vi "Editor Daten auslesen (Sub.vi).vi"(0 "Daten":string, 1 "Formatierung+Namen":string="%d", 2 "Modulname":string, 5 "Zykluslängen Namen":string) -> (6 "Zykluslänge 1":dbl, 7 "Zykluslänge 2":dbl, 8 "1":dbl[][](array[numeric]), 9 "10":dbl[][](array[numeric]), 10 "Z 1":string, 11 "Z 10":string, 12 "2":dbl[][](array[numeric]), 13 "9":dbl[][](array[numeric]), 14 "Z 2":string, 15 "Z 9":string, 16 "3":dbl[][](array[numeric]), 17 "8":dbl[][](array[numeric]), 18 "Z 3":string, 19 "Z 8":string, 20 "4":dbl[][](array[numeric]), 21 "Z 4":string, 22 "5":dbl[][](array[numeric]), 23 "Z5":string, 24 "6":dbl[][](array[numeric]), 25 "Z 6":string, 26 "7":dbl[][](array[numeric]), 27 "Z 7":string)   [LabVIEW 2010]
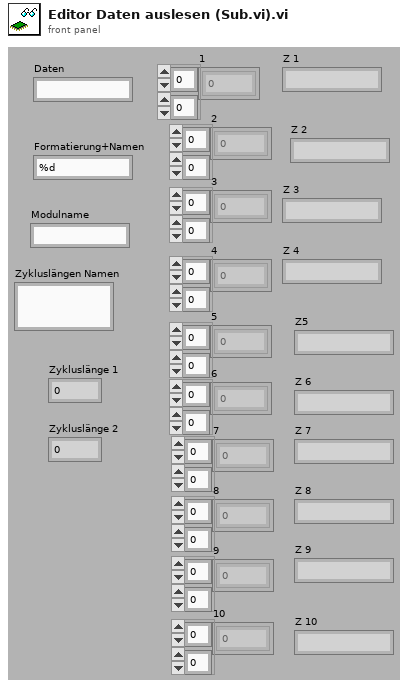
[diagram p1: front panel]
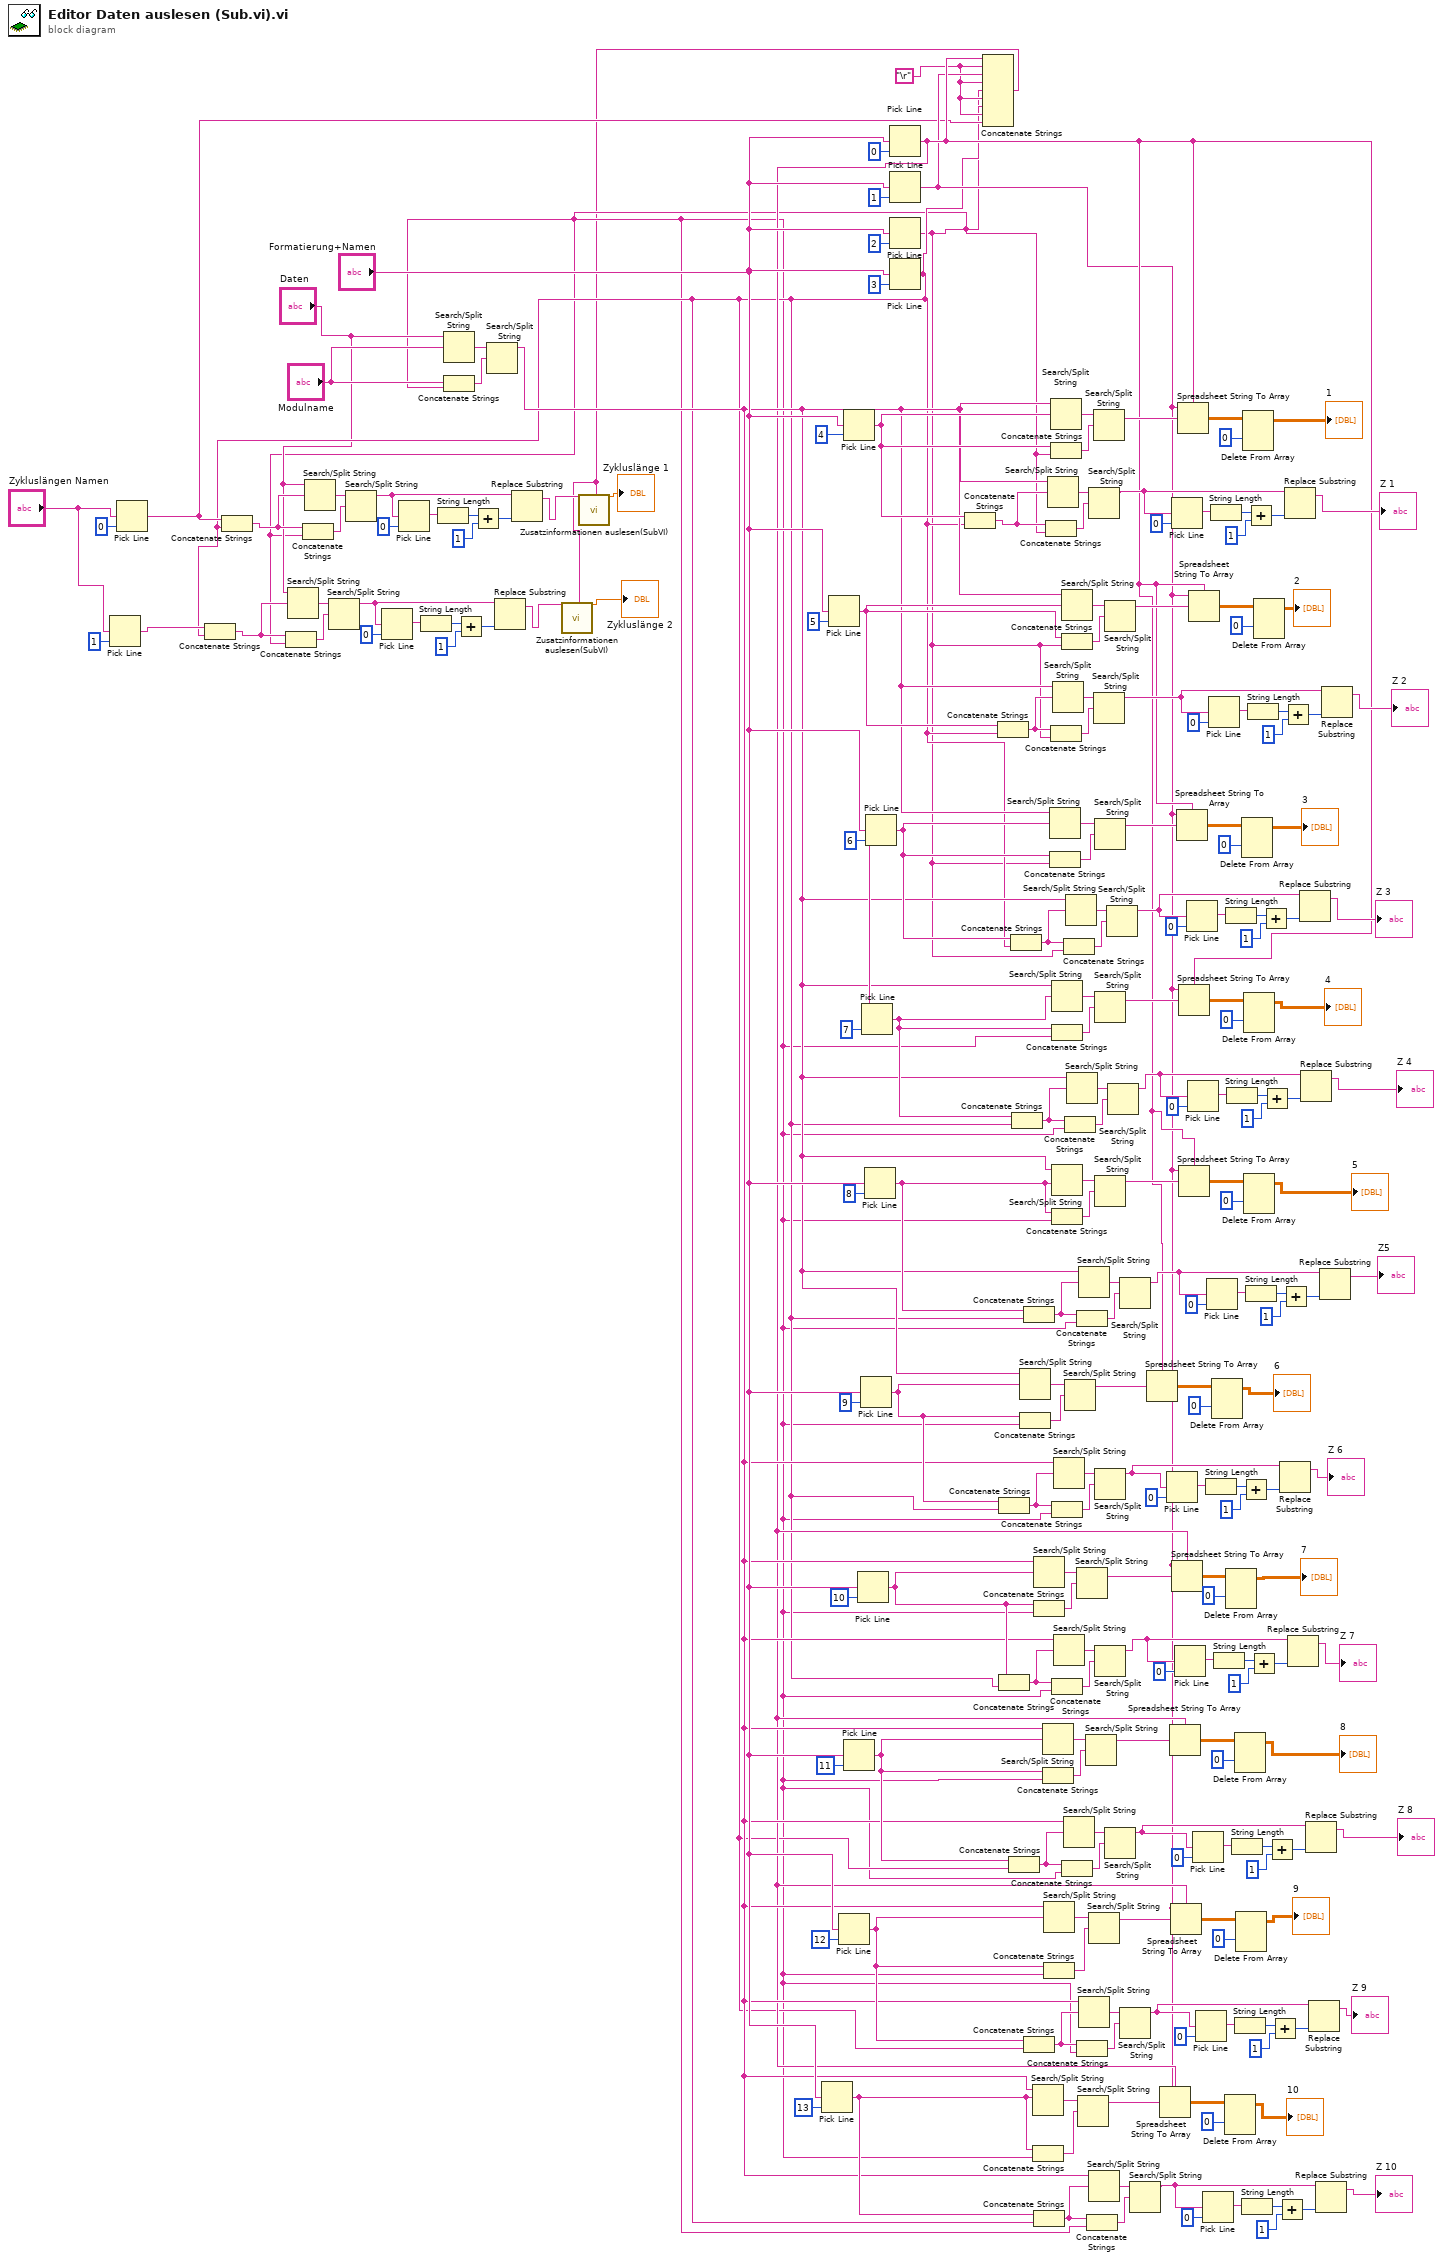
[diagram p0: block diagram]
diagram:
  w29 = "\r"
  n1 = Pick Line(multi-line string="Zykluslängen Namen", line index=1 ("Zeilenindex")) -> (output string=w5:string)  [unwired: 1 in]
  n2 = Pick Line(multi-line string="Zykluslängen Namen", line index=0 ("Zeilenindex")) -> (output string=w19:string)  [unwired: 1 in]
  n3 = Search/Split String(string="Daten", search string/char (-)="Modulname") -> (match + rest of string=w37:string)  [unwired: 1 in, 2 out]
  n4 = Pick Line(multi-line string="Formatierung+Namen", line index=13 ("Zeilenindex")) -> (output string=w110:string)  [unwired: 1 in]
  n5 = Pick Line(multi-line string="Formatierung+Namen", line index=5 ("Zeilenindex")) -> (output string=w118:string)  [unwired: 1 in]
  n6 = Pick Line(multi-line string="Formatierung+Namen", line index=12 ("Zeilenindex")) -> (output string=w111:string)  [unwired: 1 in]
  n7 = Pick Line(multi-line string="Formatierung+Namen", line index=4 ("Zeilenindex")) -> (output string=w147:string)  [unwired: 1 in]
  n8 = Pick Line(multi-line string="Formatierung+Namen", line index=11 ("Zeilenindex")) -> (output string=w112:string)  [unwired: 1 in]
  n9 = Pick Line(multi-line string="Formatierung+Namen", line index=10 ("Zeilenindex")) -> (output string=w113:string)  [unwired: 1 in]
  n10 = Pick Line(multi-line string="Formatierung+Namen", line index=9 ("Zeilenindex")) -> (output string=w114:string)  [unwired: 1 in]
  n11 = Pick Line(multi-line string="Formatierung+Namen", line index=7 ("Zeilenindex")) -> (output string=w116:string)  [unwired: 1 in]
  n12 = Pick Line(multi-line string="Formatierung+Namen", line index=8 ("Zeilenindex")) -> (output string=w115:string)  [unwired: 1 in]
  n13 = Pick Line(multi-line string="Formatierung+Namen", line index=6 ("Zeilenindex")) -> (output string=w117:string)  [unwired: 1 in]
  n14 = Pick Line(multi-line string="Formatierung+Namen", line index=0 ("Zeilenindex")) -> (output string=w31:string)  [unwired: 1 in]
  n15 = Pick Line(multi-line string="Formatierung+Namen", line index=1 ("Zeilenindex")) -> (output string=w30:string)  [unwired: 1 in]
  n16 = Pick Line(multi-line string="Formatierung+Namen", line index=2 ("Zeilenindex")) -> (output string=w2:string)  [unwired: 1 in]
  n17 = Concatenate Strings("Modulname", w2) -> (w38:string)
  n18 = Search/Split String(string=w37, search string/char (-)=w38) -> (substring before match=w36:string)  [unwired: 1 in, 2 out]
  n19 = Pick Line(multi-line string="Formatierung+Namen", line index=3 ("Zeilenindex")) -> (output string=w4:string)  [unwired: 1 in]
  n20 = Concatenate Strings(w5, w4) -> (w15:string)
  n21 = Concatenate Strings(w19, w4) -> (w33:string)
  n22 = Concatenate Strings(w15, w2) -> (w16:string)
  n23 = Search/Split String(string="Daten", search string/char (-)=w15) -> (match + rest of string=w14:string)  [unwired: 1 in, 2 out]
  n24 = Concatenate Strings(w33, w2) -> (w34:string)
  n25 = Search/Split String(string="Daten", search string/char (-)=w33) -> (match + rest of string=w32:string)  [unwired: 1 in, 2 out]
  n26 = Search/Split String(string=w14, search string/char (-)=w16) -> (substring before match=w7:string)  [unwired: 1 in, 2 out]
  n27 = Search/Split String(string=w32, search string/char (-)=w34) -> (substring before match=w22:string)  [unwired: 1 in, 2 out]
  n28 = Pick Line(multi-line string=w7, line index=0 ("Zeilenindex")) -> (output string=w11:string)  [unwired: 1 in]
  n29 = Pick Line(multi-line string=w22, line index=0 ("Zeilenindex")) -> (output string=w26:string)  [unwired: 1 in]
  n30 = String Length(string=w11) -> (length=w10:i32)
  n31 = String Length(string=w26) -> (length=w25:i32)
  n32 = Add(x=w10, y=1) -> (x+y=w8:i32)
  n33 = Add(x=w25, y=1) -> (x+y=w23:i32)
  n34 = Replace Substring(2:w8, 5:w7) -> (1:w6:string)  [unwired: 2 in, 1 out]
  n35 = Replace Substring(2:w23, 5:w22) -> (1:w21:string)  [unwired: 2 in, 1 out]
  n36 = Concatenate Strings(w147, w4) -> (w145:string)
  n37 = Concatenate Strings(w31, w29, w30, w29, w2, w29, w4, w29, w19) -> (w1:string)
  n38 = call "Zusatzinformationen auslesen(SubVI).vi"("Zusatzinformationen"=w6, "Format+Namen"=w1) -> ("1"=→"Zykluslänge 2":dbl)  [unwired: 18 in, 7 out]
  n39 = call "Zusatzinformationen auslesen(SubVI).vi"("Zusatzinformationen"=w21, "Format+Namen"=w1) -> ("1"=→"Zykluslänge 1":dbl)  [unwired: 18 in, 7 out]
  n40 = Concatenate Strings(w118, w4) -> (w142:string)
  n41 = Concatenate Strings(w114, w4) -> (w130:string)
  n42 = Concatenate Strings(w113, w4) -> (w127:string)
  n43 = Concatenate Strings(w112, w4) -> (w124:string)
  n44 = Concatenate Strings(w117, w4) -> (w139:string)
  n45 = Concatenate Strings(w116, w4) -> (w136:string)
  n46 = Search/Split String(string=w36, search string/char (-)=w114) -> (match + rest of string=w189:string)  [unwired: 1 in, 2 out]
  n47 = Concatenate Strings(w114, w2) -> (w190:string)
  n48 = Concatenate Strings(w115, w4) -> (w133:string)
  n49 = Concatenate Strings(w111, w4) -> (w121:string)
  n50 = Search/Split String(string=w36, search string/char (-)=w110) -> (match + rest of string=w209:string)  [unwired: 1 in, 2 out]
  n51 = Concatenate Strings(w110, w2) -> (w210:string)
  n52 = Search/Split String(string=w36, search string/char (-)=w113) -> (match + rest of string=w164:string)  [unwired: 1 in, 2 out]
  n53 = Concatenate Strings(w113, w2) -> (w165:string)
  n54 = Concatenate Strings(w110, w4) -> (w109:string)
  n55 = Search/Split String(string=w36, search string/char (-)=w112) -> (match + rest of string=w169:string)  [unwired: 1 in, 2 out]
  n56 = Concatenate Strings(w112, w2) -> (w170:string)
  n57 = Search/Split String(string=w36, search string/char (-)=w111) -> (match + rest of string=w174:string)  [unwired: 1 in, 2 out]
  n58 = Concatenate Strings(w111, w2) -> (w175:string)
  n59 = Concatenate Strings(w145, w2) -> (w163:string)
  n60 = Search/Split String(string=w36, search string/char (-)=w145) -> (match + rest of string=w162:string)  [unwired: 1 in, 2 out]
  n61 = Search/Split String(string=w36, search string/char (-)=w117) -> (match + rest of string=w204:string)  [unwired: 1 in, 2 out]
  n62 = Concatenate Strings(w117, w2) -> (w205:string)
  n63 = Search/Split String(string=w36, search string/char (-)=w147) -> (match + rest of string=w194:string)  [unwired: 1 in, 2 out]
  n64 = Concatenate Strings(w147, w2) -> (w195:string)
  n65 = Concatenate Strings(w142, w2) -> (w144:string)
  n66 = Search/Split String(string=w36, search string/char (-)=w116) -> (match + rest of string=w179:string)  [unwired: 1 in, 2 out]
  n67 = Concatenate Strings(w116, w2) -> (w180:string)
  n68 = Search/Split String(string=w36, search string/char (-)=w115) -> (match + rest of string=w184:string)  [unwired: 1 in, 2 out]
  n69 = Concatenate Strings(w115, w2) -> (w185:string)
  n70 = Concatenate Strings(w130, w2) -> (w132:string)
  n71 = Concatenate Strings(w127, w2) -> (w129:string)
  n72 = Search/Split String(string=w36, search string/char (-)=w142) -> (match + rest of string=w143:string)  [unwired: 1 in, 2 out]
  n73 = Search/Split String(string=w36, search string/char (-)=w130) -> (match + rest of string=w131:string)  [unwired: 1 in, 2 out]
  n74 = Search/Split String(string=w36, search string/char (-)=w127) -> (match + rest of string=w128:string)  [unwired: 1 in, 2 out]
  n75 = Search/Split String(string=w36, search string/char (-)=w118) -> (match + rest of string=w199:string)  [unwired: 1 in, 2 out]
  n76 = Concatenate Strings(w118, w2) -> (w200:string)
  n77 = Concatenate Strings(w124, w2) -> (w126:string)
  n78 = Concatenate Strings(w139, w2) -> (w141:string)
  n79 = Search/Split String(string=w36, search string/char (-)=w124) -> (match + rest of string=w125:string)  [unwired: 1 in, 2 out]
  n80 = Concatenate Strings(w136, w2) -> (w138:string)
  n81 = Search/Split String(string=w189, search string/char (-)=w190) -> (substring before match=w191:string)  [unwired: 1 in, 2 out]
  n82 = Search/Split String(string=w36, search string/char (-)=w139) -> (match + rest of string=w140:string)  [unwired: 1 in, 2 out]
  n83 = Search/Split String(string=w36, search string/char (-)=w136) -> (match + rest of string=w137:string)  [unwired: 1 in, 2 out]
  n84 = Concatenate Strings(w133, w2) -> (w135:string)
  n85 = Search/Split String(string=w164, search string/char (-)=w165) -> (substring before match=w166:string)  [unwired: 1 in, 2 out]
  n86 = Concatenate Strings(w121, w2) -> (w123:string)
  n87 = Search/Split String(string=w209, search string/char (-)=w210) -> (substring before match=w211:string)  [unwired: 1 in, 2 out]
  n88 = Search/Split String(string=w36, search string/char (-)=w133) -> (match + rest of string=w134:string)  [unwired: 1 in, 2 out]
  n89 = Search/Split String(string=w36, search string/char (-)=w121) -> (match + rest of string=w122:string)  [unwired: 1 in, 2 out]
  n90 = Search/Split String(string=w169, search string/char (-)=w170) -> (substring before match=w171:string)  [unwired: 1 in, 2 out]
  n91 = Concatenate Strings(w109, w2) -> (w120:string)
  n92 = Search/Split String(string=w162, search string/char (-)=w163) -> (substring before match=w103:string)  [unwired: 1 in, 2 out]
  n93 = Search/Split String(string=w174, search string/char (-)=w175) -> (substring before match=w176:string)  [unwired: 1 in, 2 out]
  n94 = Search/Split String(string=w36, search string/char (-)=w109) -> (match + rest of string=w119:string)  [unwired: 1 in, 2 out]
  n95 = Search/Split String(string=w194, search string/char (-)=w195) -> (substring before match=w196:string)  [unwired: 1 in, 2 out]
  n96 = Search/Split String(string=w143, search string/char (-)=w144) -> (substring before match=w96:string)  [unwired: 1 in, 2 out]
  n97 = Search/Split String(string=w204, search string/char (-)=w205) -> (substring before match=w206:string)  [unwired: 1 in, 2 out]
  n98 = Search/Split String(string=w179, search string/char (-)=w180) -> (substring before match=w181:string)  [unwired: 1 in, 2 out]
  n99 = Search/Split String(string=w184, search string/char (-)=w185) -> (substring before match=w186:string)  [unwired: 1 in, 2 out]
  n100 = Search/Split String(string=w131, search string/char (-)=w132) -> (substring before match=w68:string)  [unwired: 1 in, 2 out]
  n101 = Search/Split String(string=w128, search string/char (-)=w129) -> (substring before match=w61:string)  [unwired: 1 in, 2 out]
  n102 = Search/Split String(string=w199, search string/char (-)=w200) -> (substring before match=w201:string)  [unwired: 1 in, 2 out]
  n103 = Search/Split String(string=w125, search string/char (-)=w126) -> (substring before match=w54:string)  [unwired: 1 in, 2 out]
  n104 = Search/Split String(string=w140, search string/char (-)=w141) -> (substring before match=w89:string)  [unwired: 1 in, 2 out]
  n105 = Search/Split String(string=w137, search string/char (-)=w138) -> (substring before match=w82:string)  [unwired: 1 in, 2 out]
  n106 = Search/Split String(string=w134, search string/char (-)=w135) -> (substring before match=w75:string)  [unwired: 1 in, 2 out]
  n107 = Search/Split String(string=w122, search string/char (-)=w123) -> (substring before match=w47:string)  [unwired: 1 in, 2 out]
  n108 = Search/Split String(string=w119, search string/char (-)=w120) -> (substring before match=w40:string)  [unwired: 1 in, 2 out]
  n109 = Spreadsheet String To Array(delimiter (Tab)=w31, format string=w30, spreadsheet string=w191) -> (array=w192:dbl[][])  [unwired: 1 in]
  n110 = Spreadsheet String To Array(delimiter (Tab)=w31, format string=w30, spreadsheet string=w211) -> (array=w212:dbl[][])  [unwired: 1 in]
  n111 = Pick Line(multi-line string=w68, line index=0 ("Zeilenindex")) -> (output string=w72:string)  [unwired: 1 in]
  n112 = Spreadsheet String To Array(delimiter (Tab)=w31, format string=w30, spreadsheet string=w171) -> (array=w172:dbl[][])  [unwired: 1 in]
  n113 = Spreadsheet String To Array(delimiter (Tab)=w31, format string=w30, spreadsheet string=w176) -> (array=w177:dbl[][])  [unwired: 1 in]
  n114 = Pick Line(multi-line string=w103, line index=0 ("Zeilenindex")) -> (output string=w107:string)  [unwired: 1 in]
  n115 = Spreadsheet String To Array(delimiter (Tab)=w31, format string=w30, spreadsheet string=w166) -> (array=w167:dbl[][])  [unwired: 1 in]
  n116 = Pick Line(multi-line string=w61, line index=0 ("Zeilenindex")) -> (output string=w65:string)  [unwired: 1 in]
  n117 = Spreadsheet String To Array(delimiter (Tab)=w31, format string=w30, spreadsheet string=w206) -> (array=w207:dbl[][])  [unwired: 1 in]
  n118 = Spreadsheet String To Array(delimiter (Tab)=w31, format string=w30, spreadsheet string=w196) -> (array=w197:dbl[][])  [unwired: 1 in]
  n119 = Spreadsheet String To Array(delimiter (Tab)=w31, format string=w30, spreadsheet string=w181) -> (array=w182:dbl[][])  [unwired: 1 in]
  n120 = Spreadsheet String To Array(delimiter (Tab)=w31, format string=w30, spreadsheet string=w186) -> (array=w187:dbl[][])  [unwired: 1 in]
  n121 = Pick Line(multi-line string=w89, line index=0 ("Zeilenindex")) -> (output string=w93:string)  [unwired: 1 in]
  n122 = Pick Line(multi-line string=w82, line index=0 ("Zeilenindex")) -> (output string=w86:string)  [unwired: 1 in]
  n123 = Spreadsheet String To Array(delimiter (Tab)=w31, format string=w30, spreadsheet string=w201) -> (array=w202:dbl[][])  [unwired: 1 in]
  n124 = Pick Line(multi-line string=w54, line index=0 ("Zeilenindex")) -> (output string=w58:string)  [unwired: 1 in]
  n125 = Pick Line(multi-line string=w47, line index=0 ("Zeilenindex")) -> (output string=w51:string)  [unwired: 1 in]
  n126 = Pick Line(multi-line string=w40, line index=0 ("Zeilenindex")) -> (output string=w44:string)  [unwired: 1 in]
  n127 = String Length(string=w72) -> (length=w71:i32)
  n128 = Pick Line(multi-line string=w75, line index=0 ("Zeilenindex")) -> (output string=w79:string)  [unwired: 1 in]
  n129 = Pick Line(multi-line string=w96, line index=0 ("Zeilenindex")) -> (output string=w100:string)  [unwired: 1 in]
  n130 = String Length(string=w107) -> (length=w106:i32)
  n131 = Delete From Array(array=w192, index (row)=0 ("Index (Zeile)")) -> (array with subset deleted=→"6":dbl[][])  [unwired: 2 in, 1 out]
  n132 = String Length(string=w65) -> (length=w64:i32)
  n133 = Delete From Array(array=w212, index (row)=0 ("Index (Zeile)")) -> (array with subset deleted=→"10":dbl[][])  [unwired: 2 in, 1 out]
  n134 = String Length(string=w93) -> (length=w92:i32)
  n135 = Delete From Array(array=w167, index (row)=0 ("Index (Zeile)")) -> (array with subset deleted=→"7":dbl[][])  [unwired: 2 in, 1 out]
  n136 = String Length(string=w86) -> (length=w85:i32)
  n137 = String Length(string=w58) -> (length=w57:i32)
  n138 = Delete From Array(array=w172, index (row)=0 ("Index (Zeile)")) -> (array with subset deleted=→"8":dbl[][])  [unwired: 2 in, 1 out]
  n139 = String Length(string=w51) -> (length=w50:i32)
  n140 = Delete From Array(array=w177, index (row)=0 ("Index (Zeile)")) -> (array with subset deleted=→"9":dbl[][])  [unwired: 2 in, 1 out]
  n141 = Add(x=w71, y=1) -> (x+y=w69:i32)
  n142 = Delete From Array(array=w207, index (row)=0 ("Index (Zeile)")) -> (array with subset deleted=→"3":dbl[][])  [unwired: 2 in, 1 out]
  n143 = String Length(string=w44) -> (length=w43:i32)
  n144 = Delete From Array(array=w197, index (row)=0 ("Index (Zeile)")) -> (array with subset deleted=→"1":dbl[][])  [unwired: 2 in, 1 out]
  n145 = Delete From Array(array=w182, index (row)=0 ("Index (Zeile)")) -> (array with subset deleted=→"4":dbl[][])  [unwired: 2 in, 1 out]
  n146 = Delete From Array(array=w187, index (row)=0 ("Index (Zeile)")) -> (array with subset deleted=→"5":dbl[][])  [unwired: 2 in, 1 out]
  n147 = Add(x=w106, y=1) -> (x+y=w104:i32)
  n148 = String Length(string=w79) -> (length=w78:i32)
  n149 = String Length(string=w100) -> (length=w99:i32)
  n150 = Add(x=w64, y=1) -> (x+y=w62:i32)
  n151 = Delete From Array(array=w202, index (row)=0 ("Index (Zeile)")) -> (array with subset deleted=→"2":dbl[][])  [unwired: 2 in, 1 out]
  n152 = Add(x=w92, y=1) -> (x+y=w90:i32)
  n153 = Add(x=w85, y=1) -> (x+y=w83:i32)
  n154 = Add(x=w57, y=1) -> (x+y=w55:i32)
  n155 = Add(x=w50, y=1) -> (x+y=w48:i32)
  n156 = Add(x=w43, y=1) -> (x+y=w41:i32)
  n157 = Replace Substring(2:w69, 5:w68) -> (1:→"Z 6":string)  [unwired: 2 in, 1 out]
  n158 = Add(x=w78, y=1) -> (x+y=w76:i32)
  n159 = Add(x=w99, y=1) -> (x+y=w97:i32)
  n160 = Replace Substring(2:w104, 5:w103) -> (1:→"Z 1":string)  [unwired: 2 in, 1 out]
  n161 = Replace Substring(2:w62, 5:w61) -> (1:→"Z 7":string)  [unwired: 2 in, 1 out]
  n162 = Replace Substring(2:w90, 5:w89) -> (1:→"Z 3":string)  [unwired: 2 in, 1 out]
  n163 = Replace Substring(2:w83, 5:w82) -> (1:→"Z 4":string)  [unwired: 2 in, 1 out]
  n164 = Replace Substring(2:w55, 5:w54) -> (1:→"Z 8":string)  [unwired: 2 in, 1 out]
  n165 = Replace Substring(2:w48, 5:w47) -> (1:→"Z 9":string)  [unwired: 2 in, 1 out]
  n166 = Replace Substring(2:w41, 5:w40) -> (1:→"Z 10":string)  [unwired: 2 in, 1 out]
  n167 = Replace Substring(2:w76, 5:w75) -> (1:→"Z5":string)  [unwired: 2 in, 1 out]
  n168 = Replace Substring(2:w97, 5:w96) -> (1:→"Z 2":string)  [unwired: 2 in, 1 out]
